vi "pp2_thread test.vi"() -> ()   [LabVIEW 2013]
panel:
  out "Boolean":bool
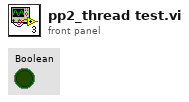
[diagram p1: front panel]
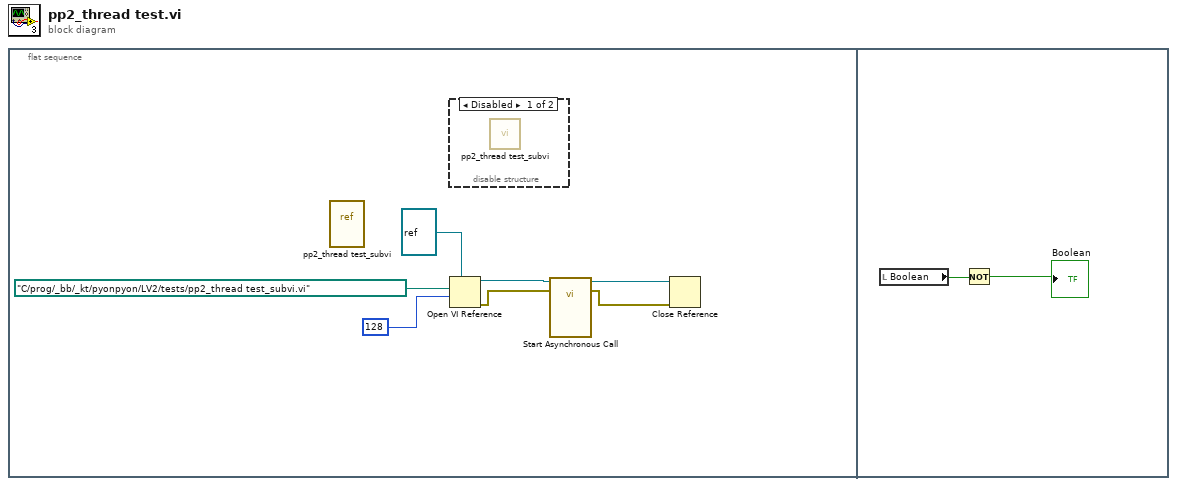
[diagram p0: block diagram]
diagram:
  n1 = flat-sequence {
    frame #0 {
      n2 = vi-ref "pp2_thread test_subvi.vi"() -> ()  [unwired: 1 out]
      n3 = disable-structure shown="Disabled" {
        frame Disabled {
          n4 = call "pp2_thread test_subvi.vi"() -> ()  [unwired: 12 in]
        }
        frame Enabled {
        }
      }
      n5 = Open VI Reference(type specifier VI Refnum (for type only)=refnum<vi> refnum, vi path=path "C:/prog/_bb/_kt/pyonpyon/LV2/tests/pp2_thread test_subvi.vi", options=128) -> (vi reference=w1:refnum<vi>, error out=w6:errorcluster)  [unwired: 3 in]
      n6 = call-by-ref "Start Asynchronous Call"(reference=w1, error in=w6) -> (reference out=w4:refnum<vi>, error out=w3:errorcluster)  [unwired: 12 in]
      n7 = Close Reference(reference=w4, error in (no error)=w3) -> ()  [unwired: 1 out]
    }
    frame #1 {
      n8 = local read "Boolean"() -> (w9:bool)
      n9 = Not(x=w9) -> (.not. x?=→"Boolean":bool)
    }
  }
